vi "sub_cost_calc.vi"(7 "decision type":enum16{"hard decision", "soft decision"}(ring), 8 "symbol map":cdb[](array[numeric]), 9 "m":i32, 10 "output bits in decimal":i32, 11 "soft symbols/ hard bits":cdb[](array[numeric])) -> (3 "cost function":dbl)   [LabVIEW 2014]
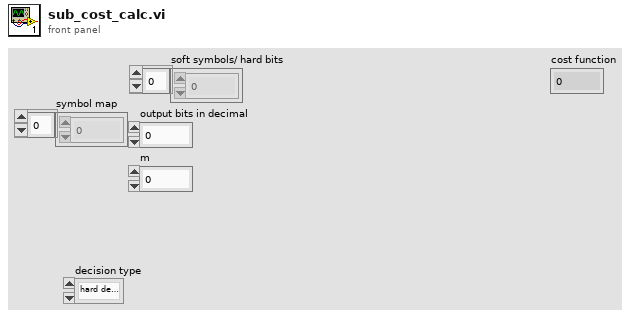
[diagram p1: front panel]
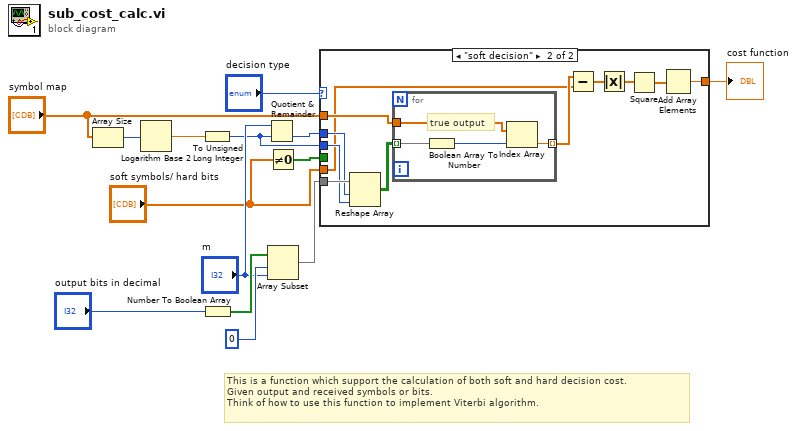
[diagram p0: block diagram]
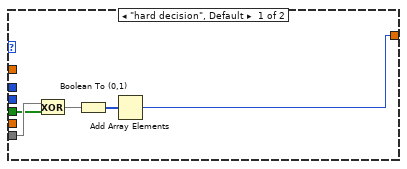
[diagram p2: hidden frame]
diagram:
  # "This is a function which support the calculation of both soft and hard decision cost.\nGiven output and received symbols or bits.\nThink of how to use this function to implement Viterbi algorithm."
  n1 = Array Size(array="symbol map") -> (size(s)=w14:i32)
  n2 = Logarithm Base 2(1:w14) -> (0:w9:dbl)
  n3 = To Unsigned Long Integer(number=w9) -> (unsigned 32bit integer=w5:u32)
  n4 = Number To Boolean Array(number="output bits in decimal") -> (Boolean array=w13:bool[])
  n5 = Quotient & Remainder(x="m", y=w5) -> (floor(x/y)=w6:u32)  [unwired: 1 out]
  n6 = Not Equal To 0?(x="soft symbols/ hard bits") -> (x != 0?=w3:bool[])
  n7 = Array Subset(array=w13, index=0, length="m") -> (w7:bool[])
  n8 = case shown="\"soft decision\"" "decision type" {
    tunnel: w7 -> [w17 w30]
    tunnel: w6 -> [_ w29]
    tunnel: w5 -> [_ w28]
    tunnel: "symbol map" -> [_ w26]
    tunnel: "soft symbols/ hard bits" -> [_ w21]
    tunnel: w3 -> [w16 _]
    tunnel: [w15 w20] -> w2
    frame "hard decision", Default {
      n9 = Exclusive Or(1:w16, 2:w17) -> (0:w19:bool[])
      n10 = Boolean To (0,1)(Boolean=w19) -> (0, 1=w18:i16[])
      n11 = Add Array Elements(numeric array=w18) -> (sum=w15:i16)
    }
    frame "soft decision" {
      n12 = Reshape Array(w30, w29, w28) -> (w27:bool[][])
      n13 = for {
        tunnel: w26 -> [w34]
        tunnel: w27 -> [w33] mode=indexing
        tunnel: [w31] -> w22 mode=indexing
        # "true output"
        n14 = Boolean Array To Number(Boolean array=w33) -> (number=w32:u32)
        n15 = Index Array(array=w34, index=w32) -> (element=w31:cdb)
      }
      n16 = Subtract(x=w22, y=w21) -> (x-y=w25:cdb[])
      n17 = Absolute Value(x=w25) -> (abs(x)=w24:dbl[])
      n18 = Square(x=w24) -> (x^2=w23:dbl[])
      n19 = Add Array Elements(numeric array=w23) -> (sum=w20:dbl)
    }
  }
  "cost function" <- w2
